vi "unknown graph.vi"(6 "Boolean":bool, 7 "Coords":T2, 8 "error in":errorcluster, 10 "DATA CLUSTER in":T1, 11 "CtlRef":refnum<vi>) -> (0 "error out":errorcluster, 2 "graph out":T3(array[cluster]))   [LabVIEW 2016]
uses:
  <vilib>/Utility/miscctls.llb/LVPoint32TypeDef.ctl
  controls/data control cluster.ctl
panel:
  out "cycle result header":string[](array[string])
  out "sequence result header":string[](array[string])
  out "sequence  Result":dbl[][](array[numeric])
  out "x-y":dbl[](array[numeric])
  out "x+y":dbl[](array[numeric])
  out "Cycle data by position":dbl[][][](array[numeric])
  out "subarray":dbl[](array[numeric])
  out "Yerror 2":dbl[](array[numeric])
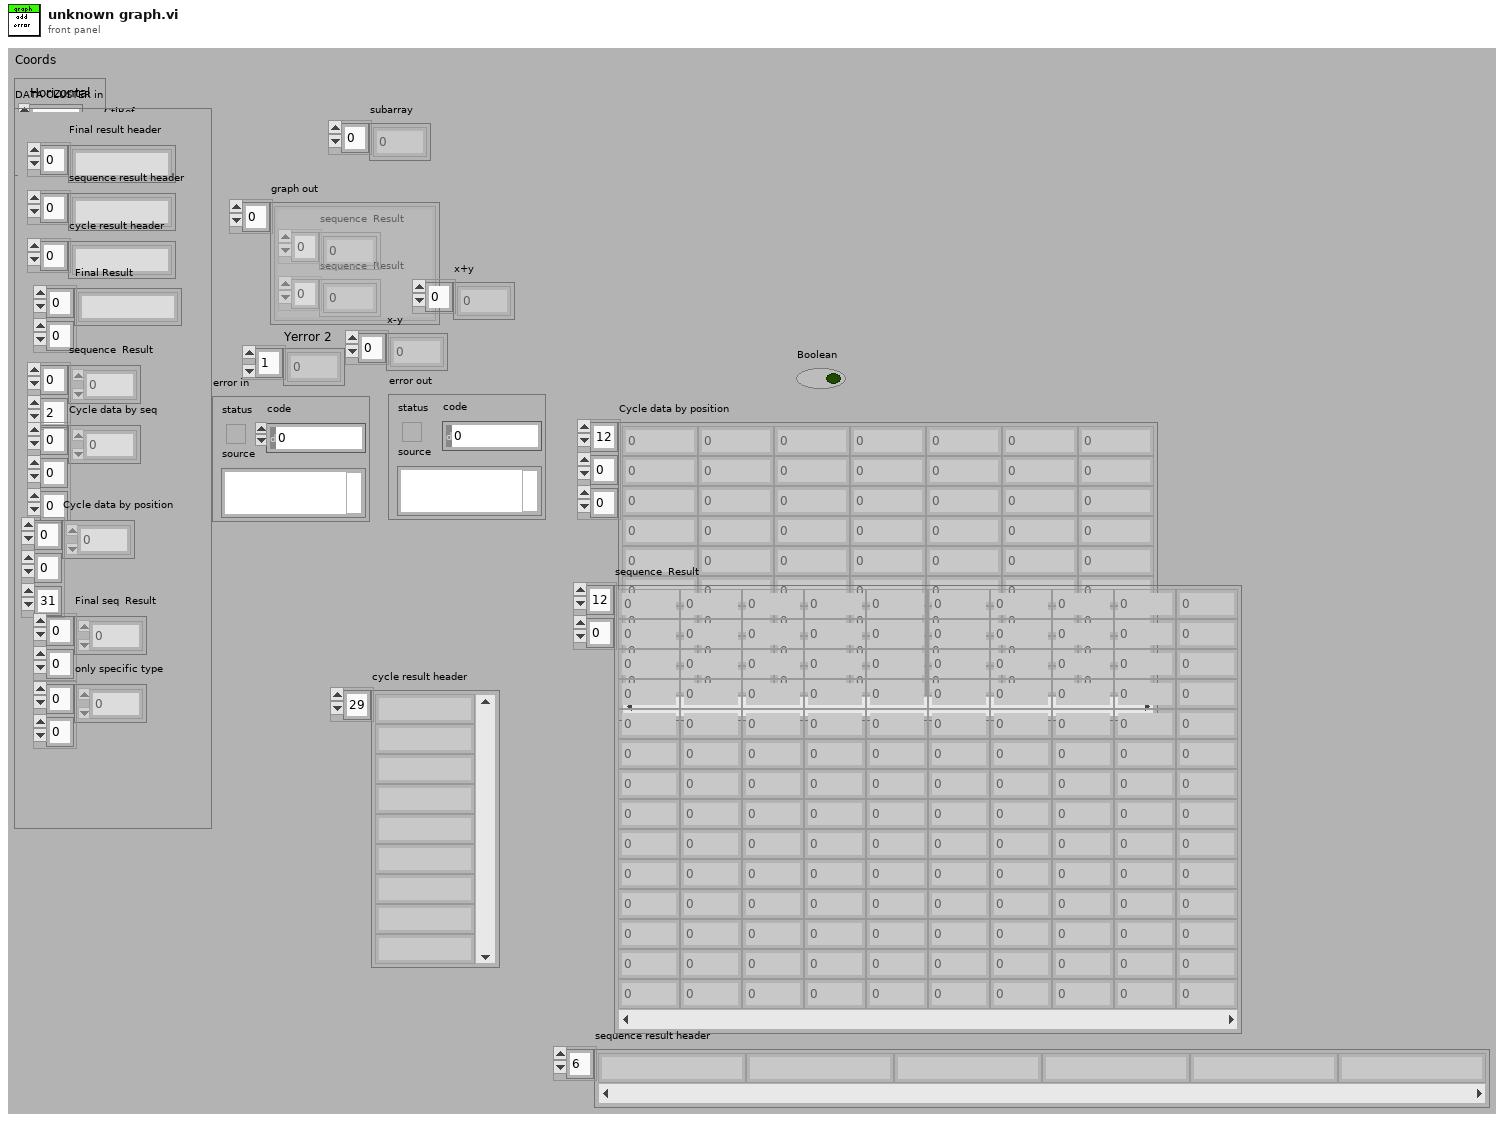
[diagram p1: front panel]
types:
  T1 = typedef "data control cluster.ctl" = cluster{"Final result header":string[], "sequence result header":string[], "cycle result header ":string[], "Final Result":string[][], "sequence  Result":dbl[][], "Cycle data by seq":dbl[][][], "Cycle data by position":dbl[][][], "Final seq  Result":dbl[][], "only specific type":dbl[][]}
  T2 = typedef "LVPoint32TypeDef.ctl" = cluster{"Horizontal":i32, "Vertical":i32}
  T3 = cluster{"sequence  Result":dbl[], "sequence  Result":dbl[]}[]
  T4 = cluster{"array w/ subset deleted":dbl[], "array w/ subset deleted":dbl[]}
  T5 = cluster{"array w/ subset deleted":dbl[], "array w/ subset deleted":dbl[]}[]
  T6 = cluster{"Cycle data by seq":dbl[], "Cycle data by seq":dbl[]}
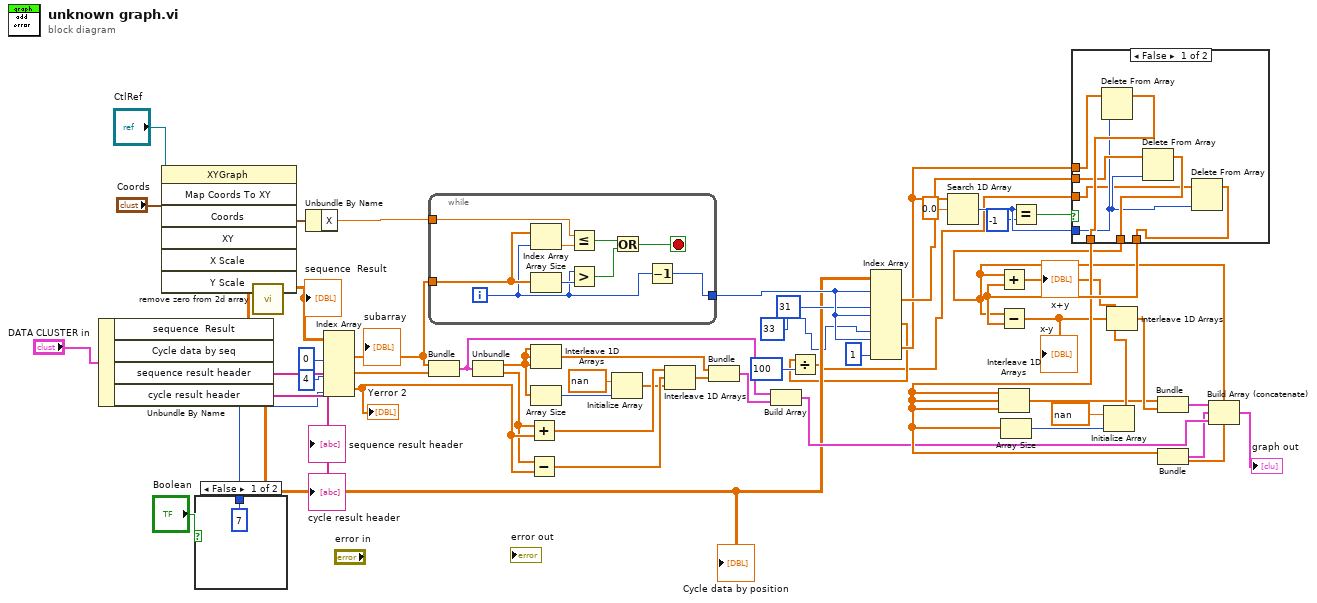
[diagram p0: block diagram]
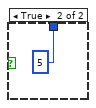
[diagram p2: hidden frame]
diagram:
  n1 = Unbundle By Name("DATA CLUSTER in") -> ("sequence  Result"=w5:dbl[][], "Cycle data by seq"=w11:dbl[][][], "sequence result header"=→"sequence result header":string[], "cycle result header"=→"cycle result header":string[])
  "Cycle data by position" <- w11
  n2 = invoke class="XYGraph" method="Map Coords To XY"(reference="CtlRef", "Coords"="Coords") -> ("XY"=w30:cluster{"X":dbl, "Y":dbl})  [unwired: 5 in, 6 out]
  n3 = case shown="False" "Boolean" {
    tunnel: [7 ("index (col)") 5 ("index (col)")] -> w1
    frame False {
    }
    frame True {
    }
  }
  n4 = call "remove zero from 2d array.vi"("Cycle data by seq"=w5) -> ("array w/ subset deleted"=w4:dbl[][])  [unwired: 10 in]
  "sequence  Result" <- w4
  n5 = Unbundle By Name(w30) -> ("X"=w31:dbl)
  n6 = Index Array(array=w4, index (col) #1=0 ("disabled index (col)"), index (col) #2=4 ("index (col)"), index (col) #3=w1) -> (element #1=w32:dbl[], element #2=w18:dbl[], element #3=w17:dbl[])  [unwired: 3 in]
  "Yerror 2" <- w17
  "subarray" <- w32
  n7 = while {
    tunnel: w31 -> [w62]
    tunnel: w32 -> [w66]
    tunnel: [w58] -> w35
    i -> [w59]
    stop <- w63 stop-if-true
    n8 = Index Array(array=w66, index=w59) -> (element=w61:dbl)
    n9 = Array Size(array=w66) -> (size(s)=w65:i32)
    n10 = Less Or Equal?(x=w62, y=w61) -> (x <= y?=w60:bool)
    n11 = Greater?(x=w59, y=w65) -> (0:w64:bool)
    n12 = Or(x=w60, y=w64) -> (x .or. y?=w63:bool)
    n13 = Decrement(x=w59) -> (x-1=w58:i32)
  }
  n14 = Bundle("array w/ subset deleted"=w32, "array w/ subset deleted"=w18) -> (w19:T4)  [unwired: 1 in]
  n15 = Unbundle(w19) -> ("array w/ subset deleted"=w12:dbl[], "array w/ subset deleted"=w13:dbl[])
  n16 = Add(x=w13, y=w17) -> (x+y=w25:dbl[])
  n17 = Subtract(x=w13, y=w17) -> (x-y=w24:dbl[])
  n18 = Interleave 1D Arrays(w12, w12, w12) -> (w26:dbl[])
  n19 = Array Size(array=w12) -> (size(s)=w23:i32)
  n20 = Initialize Array(nan ("element"), w23) -> (w22:dbl[])
  n21 = Interleave 1D Arrays(w25, w24, w22) -> (w27:dbl[])
  n22 = Bundle(w26, w27) -> (w20:cluster{dbl[], dbl[]})  [unwired: 1 in]
  n23 = Build Array(w19, w20) -> (w45:T5)
  n24 = Index Array(array=w11, index (dim 0) #1=w35, index (dim 2) #1=31 ("disabled index (col)"), index (dim 0) #2=w35, index (dim 2) #2=33 ("index (col)"), index (dim 0) #3=w35, index (dim 2) #3=1 ("index (col)")) -> (element #1=w51:dbl[], element #2=w7:dbl[], element #3=w50:dbl[])  [unwired: 3 in]
  n25 = Divide(x=w7, y=100) -> (x/y=w6:dbl[])
  n26 = Search 1D Array(1D array=w50, element=0.0) -> (index of element=w55:i32)  [unwired: 1 in]
  n27 = Equal?(x=w55, y=-1) -> (x = y?=w49:bool)
  n28 = case shown="False" w49 {
    tunnel: w51 -> [w71 w76]
    tunnel: w50 -> [w73 w75]
    tunnel: [w70 w76] -> w52
    tunnel: [w72 w75] -> w53
    tunnel: w6 -> [w68 w74]
    tunnel: [w67 w74] -> w54
    tunnel: w55 -> [w69 _]
    frame False {
      n29 = Delete From Array(array=w73, index=w69) -> (array with subset deleted=w72:dbl[])  [unwired: 1 in, 1 out]
      n30 = Delete From Array(array=w71, index=w69) -> (array with subset deleted=w70:dbl[])  [unwired: 1 in, 1 out]
      n31 = Delete From Array(array=w68, index=w69) -> (array with subset deleted=w67:dbl[])  [unwired: 1 in, 1 out]
    }
    frame True {
    }
  }
  n32 = Add(x=w52, y=w54) -> (x+y=w36:dbl[])
  "x+y" <- w36
  n33 = Subtract(x=w52, y=w54) -> (x-y=w37:dbl[])
  "x-y" <- w37
  n34 = Interleave 1D Arrays(w53, w53, w53) -> (w39:dbl[])
  n35 = Array Size(array=w53) -> (size(s)=w38:i32)
  n36 = Initialize Array(nan ("element"), w38) -> (w41:dbl[])
  n37 = Interleave 1D Arrays(w36, w37, w41) -> (w42:dbl[])
  n38 = Bundle(w39, w42) -> (w43:cluster{dbl[], dbl[]})  [unwired: 1 in]
  n39 = Bundle("Cycle data by seq"=w53, "Cycle data by seq"=w52) -> (w44:T6)  [unwired: 1 in]
  n40 = Build Array (concatenate)(w43, w44, w45) -> (→"graph out":T5)
